vi "FTW-CodeGen-Image.vi"(0 "State In":T1, 5 "XRef":refnum<vi>) -> (4 "Image":picture)   [LabVIEW 2014, in "FTW-SQLite-Insert.xnode"]
uses:
  FTW-SQLite-Insert.xnode
  FTW-CodeGen-State.ctl
panel:
  # "Inputs"
  # "Outputs"
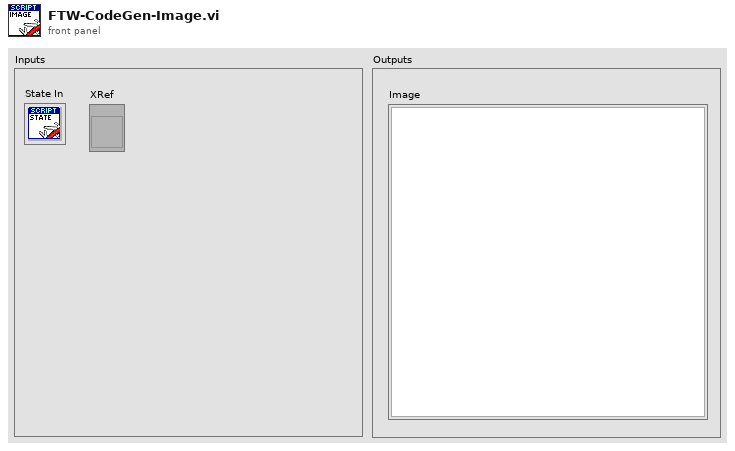
[diagram p1: front panel]
types:
  T1 = typedef "FTW-SQLite-Insert.xnode/FTW-CodeGen-State.ctl" = cluster{"Dummy":i32}
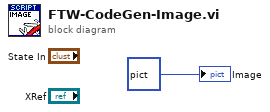
[diagram p0: block diagram]
diagram:
  "Image" <- picture bytes[3232] ("Picture")
